vi "Set Default Value.vi"(9 "Default C++ Value":string, 10 "Control Ref":refnum<vi>, 11 "Number Writer in":refnum<class "Number Writer.lvclass">) -> (1 "LabVIEW Default String":string, 2 "Control Ref Dup":refnum<vi>, 3 "Number Writer out":refnum<class "Number Writer.lvclass">)   [LabVIEW 2013, in "Number Writer.lvclass"]
doc: "Copyright (c) 2016 Sze Howe Koh\n\nThis Source Code Form is subject to the terms of the Mozilla Public License, v. 2.0. If a copy of the MPL was not distributed with this file, You can obtain one at http://mozilla.org/MPL/2.0/."
uses:
  Number Writer.lvclass
  Number Writer.lvclass/Number Writer.ctl
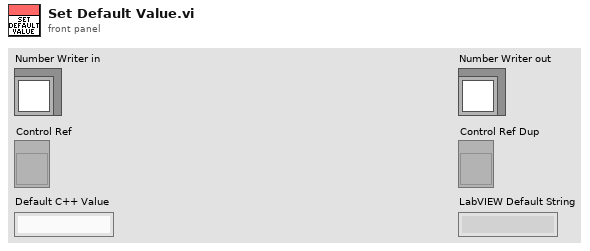
[diagram p1: front panel]
types:
  T1 = typedef "Number Writer.lvclass/Numeric Type.ctl" = enum16{"I8", "I16", "I32", "I64", "U8", "U16", "U32", "U64", "SGL", "DBL", "PTR INT", "PTR UINT"}
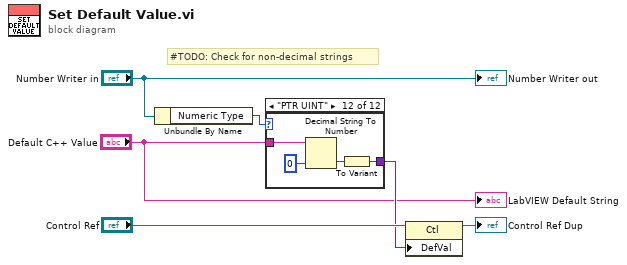
[diagram p0: block diagram]
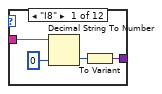
[diagram p2: hidden frame]
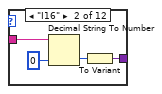
[diagram p3: hidden frame]
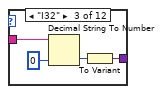
[diagram p4: hidden frame]
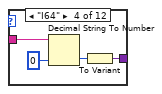
[diagram p5: hidden frame]
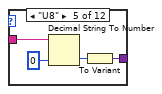
[diagram p6: hidden frame]
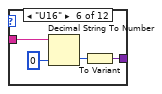
[diagram p7: hidden frame]
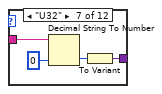
[diagram p8: hidden frame]
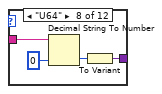
[diagram p9: hidden frame]
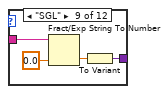
[diagram p10: hidden frame]
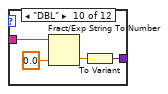
[diagram p11: hidden frame]
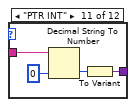
[diagram p12: hidden frame]
diagram:
  # "#TODO: Check for non-decimal strings"
  n1 = Unbundle By Name("Number Writer in") -> ("Numeric Type"=w3:T1)
  n2 = case shown="\"PTR UINT\"" w3 {
    tunnel: "Default C++ Value" -> [w10 w14 w18 w22 w26 w30 w34 w38 w42 w46 w50 w54]
    tunnel: [w7 w11 w15 w19 w23 w27 w31 w35 w39 w43 w47 w51] -> w2
    frame "I8" {
      n3 = Decimal String To Number(string=w10, default (0L)=i8 0) -> (number=w8:i8)  [unwired: 1 in, 1 out]
      n4 = To Variant(anything=w8) -> (Variant=w7:variant)
    }
    frame "I16" {
      n5 = Decimal String To Number(string=w14, default (0L)=i16 0) -> (number=w12:i16)  [unwired: 1 in, 1 out]
      n6 = To Variant(anything=w12) -> (Variant=w11:variant)
    }
    frame "I32" {
      n7 = Decimal String To Number(string=w18, default (0L)=0) -> (number=w16:i32)  [unwired: 1 in, 1 out]
      n8 = To Variant(anything=w16) -> (Variant=w15:variant)
    }
    frame "I64" {
      n9 = Decimal String To Number(string=w22, default (0L)=i64 0) -> (number=w20:i64)  [unwired: 1 in, 1 out]
      n10 = To Variant(anything=w20) -> (Variant=w19:variant)
    }
    frame "U8" {
      n11 = Decimal String To Number(string=w26, default (0L)=u8 0) -> (number=w24:u8)  [unwired: 1 in, 1 out]
      n12 = To Variant(anything=w24) -> (Variant=w23:variant)
    }
    frame "U16" {
      n13 = Decimal String To Number(string=w30, default (0L)=u16 0) -> (number=w28:u16)  [unwired: 1 in, 1 out]
      n14 = To Variant(anything=w28) -> (Variant=w27:variant)
    }
    frame "U32" {
      n15 = Decimal String To Number(string=w34, default (0L)=u32 0) -> (number=w32:u32)  [unwired: 1 in, 1 out]
      n16 = To Variant(anything=w32) -> (Variant=w31:variant)
    }
    frame "U64" {
      n17 = Decimal String To Number(string=w38, default (0L)=u64 0) -> (number=w36:u64)  [unwired: 1 in, 1 out]
      n18 = To Variant(anything=w36) -> (Variant=w35:variant)
    }
    frame "SGL" {
      n19 = Fract/Exp String To Number(string=w42, default (0 dbl)=sgl 0.0) -> (number=w40:sgl)  [unwired: 2 in, 1 out]
      n20 = To Variant(anything=w40) -> (Variant=w39:variant)
    }
    frame "DBL" {
      n21 = Fract/Exp String To Number(string=w46, default (0 dbl)=0.0) -> (number=w44:dbl)  [unwired: 2 in, 1 out]
      n22 = To Variant(anything=w44) -> (Variant=w43:variant)
    }
    frame "PTR INT" {
      n23 = Decimal String To Number(string=w50, default (0L)=i64 0) -> (number=w48:i64)  [unwired: 1 in, 1 out]
      n24 = To Variant(anything=w48) -> (Variant=w47:variant)
    }
    frame "PTR UINT" {
      n25 = Decimal String To Number(string=w54, default (0L)=u64 0) -> (number=w52:u64)  [unwired: 1 in, 1 out]
      n26 = To Variant(anything=w52) -> (Variant=w51:variant)
    }
  }
  n27 = property class="Ctl"(reference="Control Ref", "DefVal"=w2) -> (reference out=→"Control Ref Dup":refnum<vi>)  [unwired: 1 in, 1 out]
  "Number Writer out" <- "Number Writer in"
  "LabVIEW Default String" <- "Default C++ Value"
